vi "sequential on_off.vi"() -> ()   [LabVIEW 2018]
doc: "Manually blink and LED attached to a digital output channel of a LINX device by clicking and LED control in LabVIEW."
uses:
  <vilib>/MakerHub/LINX/Public/Peripherals/Digital/Digital Write 1 Chan.vi
  <vilib>/MakerHub/LINX/Public/Peripherals/Digital/Digital Write N Chans.vi
  <vilib>/MakerHub/LINX/Private/Local IO/LinxDigitalWrite.vi
  <vilib>/MakerHub/LINX/Public/Utilities/Check Channel.vi
  <vilib>/MakerHub/LINX/Public/Utilities/Open Serial.vi
  <vilib>/MakerHub/LINX/Private/Utilties/Generate Error.vi
  <vilib>/MakerHub/LINX/LMH-LINX.lvlib
panel:
  out "ch_4":bool
  out "ch_3":bool
  out "ch_2":bool
  out "ch_1":bool
  in  "Delay (ms)":dbl
  in  "Chnl_4":bool
  in  "Chnl_3":bool
  in  "Chnl_2":bool
  in  "Chnl_1":bool
  in  "Reset valves":bool
  out "id_8":bool
  out "id_7":bool
  out "id_6":bool
  out "id_5":bool
  out "id_4":bool
  out "id_3":bool
  out "id_2":bool
  out "id_1":bool
  in  "stop":bool
  in  "Valve 8":bool
  in  "Valve 7":bool
  in  "Valve 6":bool
  in  "Valve 5":bool
  in  "Valve 4":bool
  in  "Valve 3":bool
  in  "Valve 2":bool
  in  "Valve_1":bool
  in  "Serial Port":refnum<visa-resource-name>
  # "Manual Control:"
  # "LINX Device Settings"
  # "Sequential Control:"
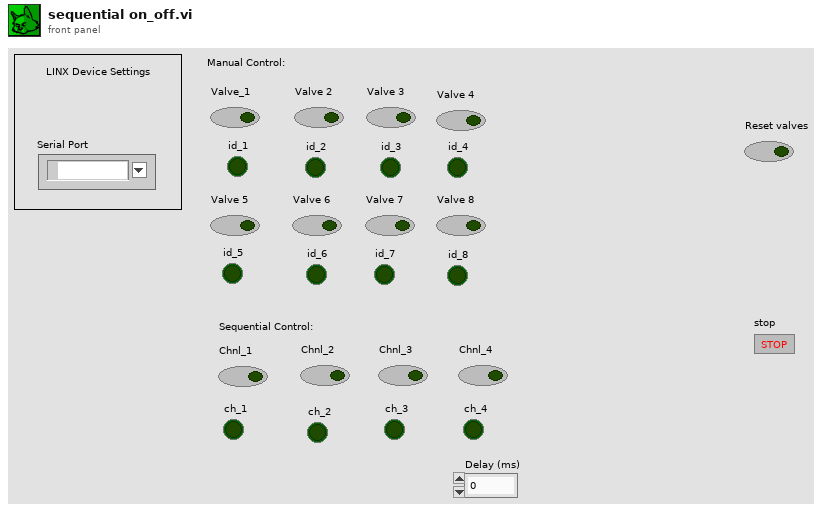
[diagram p1: front panel]
types:
  T1 = typedef "LMH-LINX.lvlib/LINX Ref.ctl" = cluster{"IO":T2, "Interface":T3, "LINX Device Config":T4}
  T2 = typedef "LMH-LINX.lvlib/Platform.ctl" = enum16{"Remote", "Local"}
  T3 = typedef "LMH-LINX.lvlib/Interface.ctl" = enum16{"Serial", "TCP"}
  T4 = typedef "LMH-LINX.lvlib/Device.lvlib/LINX Device Config.ctl" = cluster{"Interface":T3, "COM Port":refnum<visa-resource-name>, "TCP Configuration":T5, "Device Family":u8, "Device ID":u8, "Device Name":string, "TCP Ref":refnum<k5>, "Channels":T6}
  T5 = typedef "LMH-LINX.lvlib/Device.lvlib/TCP Config.ctl" = cluster{"IP Address":string, "Port":u16}
  T6 = typedef "LMH-LINX.lvlib/Channels.ctl" = cluster{"DI":u8[], "DO":u8[], "AI":u8[], "AO":u8[], "PWM":u8[], "QE":u8[], "UART":u8[], "I2C 2":u8[], "SPI":u8[], "CAN":u8[], "Servo":u8[], "AI Ref (V)":dbl, "AI Resolution (Bits)":u8, "AO Ref (V)":dbl, "AO Resolution (Bits)":u8}
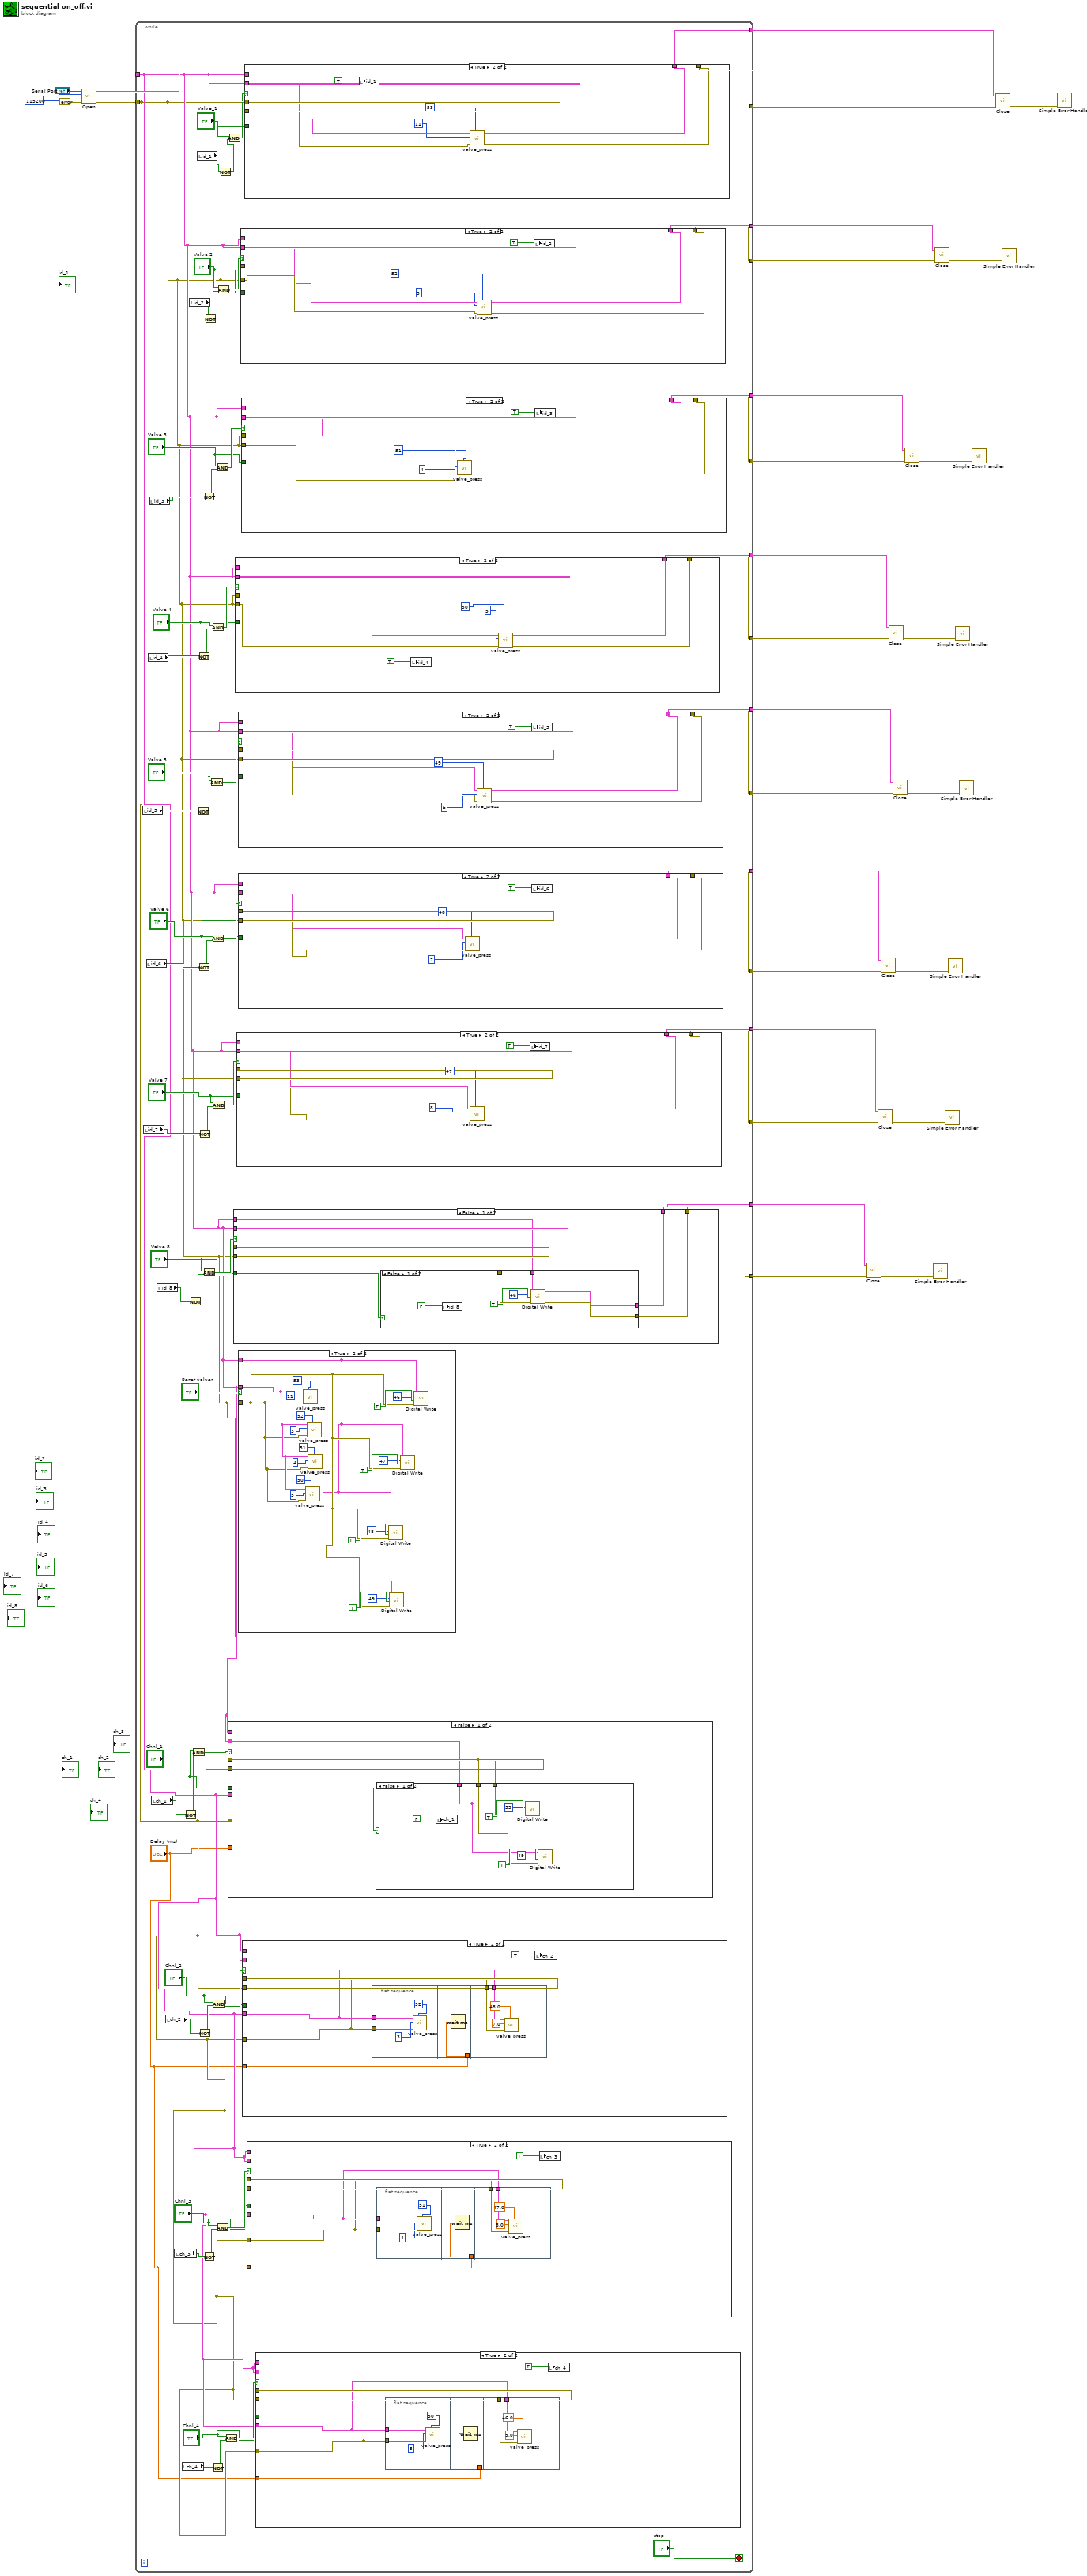
[diagram p0: block diagram]
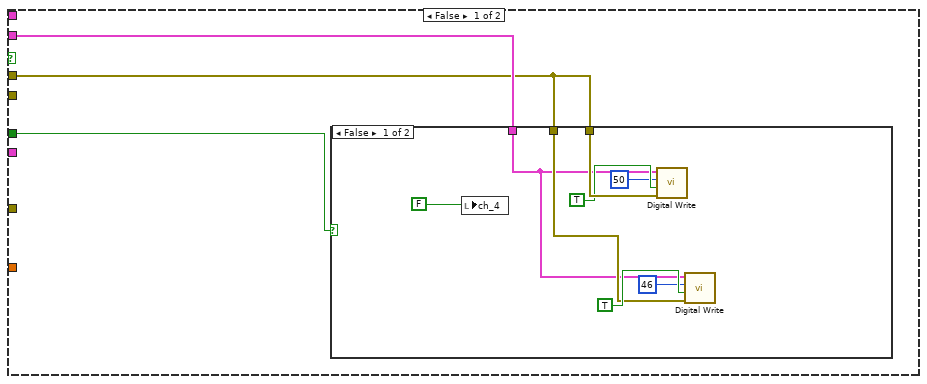
[diagram p2: hidden frame]
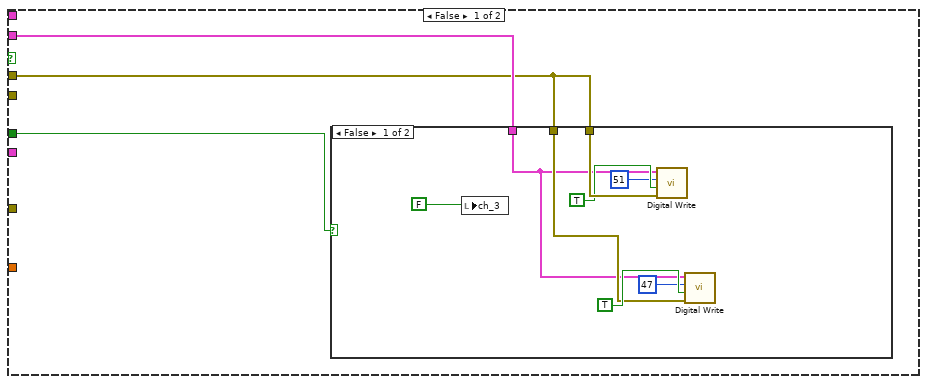
[diagram p4: hidden frame]
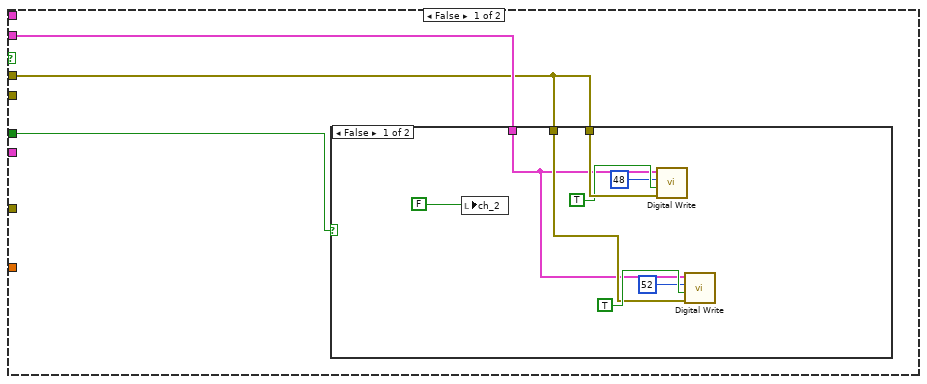
[diagram p6: hidden frame]
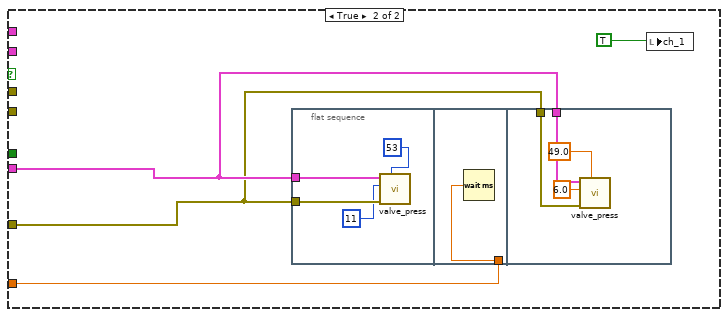
[diagram p9: hidden frame]
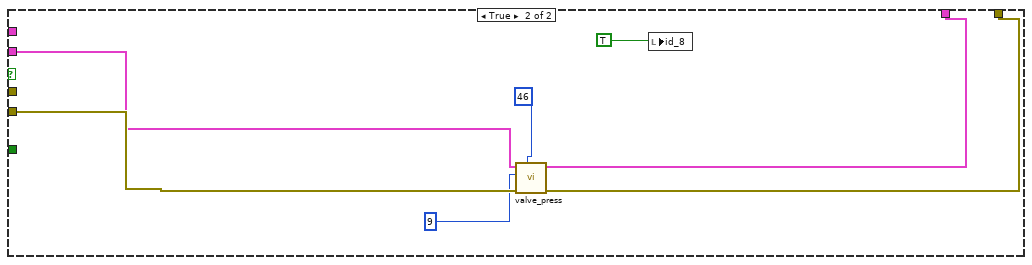
[diagram p12: hidden frame]
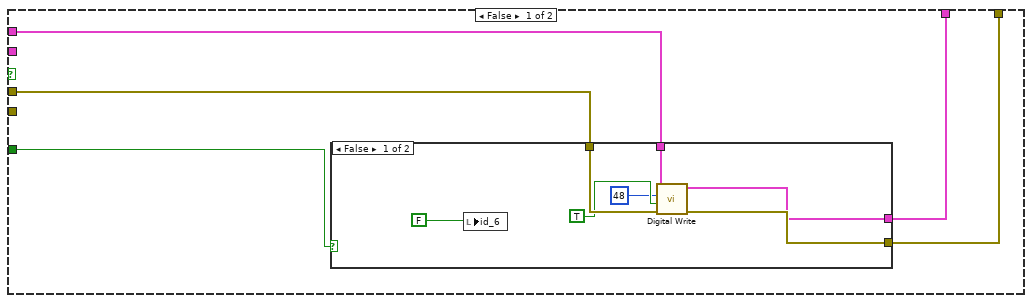
[diagram p13: hidden frame]
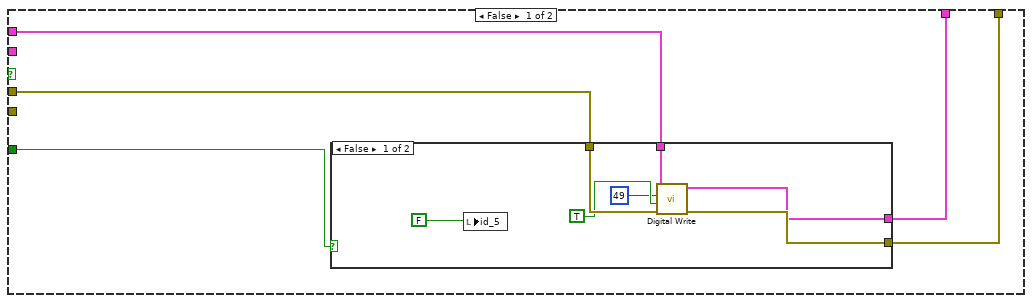
[diagram p15: hidden frame]
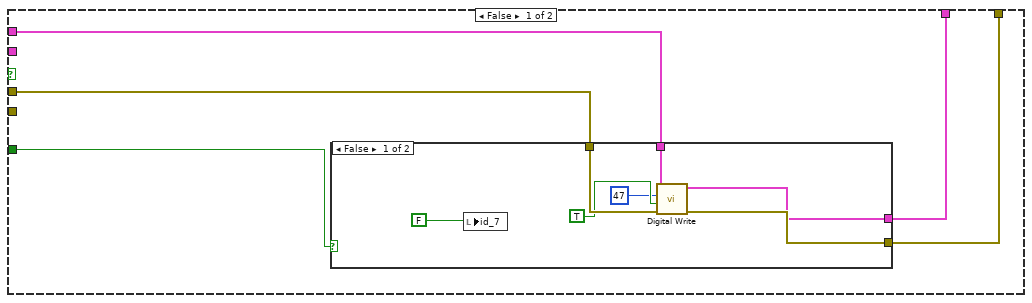
[diagram p17: hidden frame]
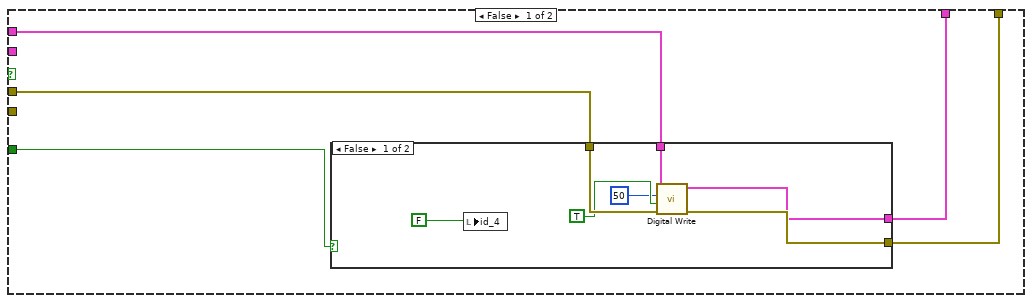
[diagram p19: hidden frame]
diagram:
  n1 = call-poly <vilib>:"Open.vi"("Error In"=errorcluster {"status"=FALSE, "code"=0, "source"=""}, "Baud Rate Override"=u32 115200, "Serial Port"="Serial Port") -> ("Error Out"=w25:errorcluster, "LINX Resource"=w26:T1)  [unwired: 6 in, 1 out]
  n2 = while {
    tunnel: w26 -> [w35]
    tunnel: w25 -> [w34]
    tunnel: [w97] -> w24
    tunnel: [w96] -> w23
    tunnel: [w92] -> w21
    tunnel: [w91] -> w14
    tunnel: [w90] -> w13
    tunnel: [w89] -> w12
    tunnel: [w88] -> w11
    tunnel: [w87] -> w10
    tunnel: [w86] -> w9
    tunnel: [w85] -> w8
    tunnel: [w84] -> w7
    tunnel: [w83] -> w6
    tunnel: [w82] -> w5
    tunnel: [w81] -> w4
    tunnel: [w50] -> w3
    tunnel: [w73] -> w2
    stop <- "stop" stop-if-true
    n3 = local read "id_5"() -> (w68:bool)
    n4 = local read "id_7"() -> (w66:bool)
    n5 = local read "id_6"() -> (w67:bool)
    n6 = local read "id_4"() -> (w69:bool)
    n7 = local read "id_3"() -> (w70:bool)
    n8 = local read "ch_1"() -> (w49:bool)
    n9 = local read "id_8"() -> (w65:bool)
    n10 = local read "ch_2"() -> (w45:bool)
    n11 = local read "ch_3"() -> (w38:bool)
    n12 = local read "ch_4"() -> (w32:bool)
    n13 = Not(x=w49) -> (.not. x?=w48:bool)
    n14 = Not(x=w65) -> (.not. x?=w64:bool)
    n15 = local read "id_2"() -> (w78:bool)
    n16 = And(x="Chnl_1", y=w48) -> (x .and. y?=w47:bool)
    n17 = Not(x=w68) -> (.not. x?=w58:bool)
    n18 = local read "id_1"() -> (w94:bool)
    n19 = Not(x=w69) -> (.not. x?=w72:bool)
    n20 = Not(x=w67) -> (.not. x?=w60:bool)
    n21 = Not(x=w66) -> (.not. x?=w62:bool)
    n22 = Not(x=w45) -> (.not. x?=w44:bool)
    n23 = Not(x=w70) -> (.not. x?=w76:bool)
    n24 = And(x="Valve 8", y=w64) -> (x .and. y?=w63:bool)
    n25 = Not(x=w38) -> (.not. x?=w41:bool)
    n26 = Not(x=w78) -> (.not. x?=w79:bool)
    n27 = And(x="Valve 5", y=w58) -> (x .and. y?=w57:bool)
    n28 = And(x="Valve 4", y=w72) -> (x .and. y?=w71:bool)
    n29 = And(x="Valve 6", y=w60) -> (x .and. y?=w59:bool)
    n30 = Not(x=w32) -> (.not. x?=w37:bool)
    n31 = And(x="Valve 7", y=w62) -> (x .and. y?=w61:bool)
    n32 = And(x="Chnl_2", y=w44) -> (x .and. y?=w43:bool)
    n33 = And(x="Valve 3", y=w76) -> (x .and. y?=w75:bool)
    n34 = And(x="Chnl_3", y=w41) -> (x .and. y?=w40:bool)
    n35 = And(x="Valve 2", y=w79) -> (x .and. y?=w80:bool)
    n36 = Not(x=w94) -> (.not. x?=w93:bool)
    n37 = And(x="Chnl_4", y=w37) -> (x .and. y?=w36:bool)
    n38 = And(x="Valve_1", y=w93) -> (x .and. y?=w95:bool)
    n39 = case shown="False" w47 {
      tunnel: w35 -> [w172 _]
      tunnel: w34 -> [_ _]
      tunnel: "Chnl_1" -> [w173 _]
      tunnel: w34 -> [w171 _]
      tunnel: w35 -> [_ _]
      tunnel: w34 -> [_ w183]
      tunnel: w35 -> [_ w184]
      tunnel: "Delay (ms)" -> [_ w185]
      frame False {
        n40 = case shown="False" w173 {
          tunnel: w171 -> [w181 _]
          tunnel: w172 -> [w174 _]
          tunnel: w171 -> [w175 _]
          frame False {
            n41 = local write "ch_1"(FALSE) -> ()
            n42 = call-poly <vilib>:"Digital Write.vi"("Error In"=w181, "Output Value"=TRUE, "DO Channel"=u8 53, "LINX Resource"=w174) -> ()  [unwired: 6 in, 2 out]
            n43 = call-poly <vilib>:"Digital Write.vi"("Error In"=w175, "Output Value"=TRUE, "DO Channel"=u8 49, "LINX Resource"=w174) -> ()  [unwired: 6 in, 2 out]
          }
          frame True {
          }
        }
      }
      frame True {
        n44 = flat-sequence {
          tunnel: w183 -> [w188]
          tunnel: w184 -> [w186]
          tunnel: w185 -> [w190]
          tunnel: w184 -> [w194]
          tunnel: w183 -> [w193]
          frame #0 {
            n45 = call "valve_press.vi"("power"=53, "error in (no error)"=w188, "trigger"=11, "LINX Resource in"=w186) -> ()  [unwired: 6 in, 2 out]
          }
          frame #1 {
            n46 = Wait (ms)(milliseconds to wait=w190) -> ()  [unwired: 1 out]
          }
          frame #2 {
            n47 = call "valve_press.vi"("power"=49.0, "error in (no error)"=w193, "trigger"=6.0, "LINX Resource in"=w194) -> ()  [unwired: 6 in, 2 out]
          }
        }
        n48 = local write "ch_1"(TRUE) -> ()
      }
    }
    n49 = case shown="False" w63 {
      tunnel: w35 -> [_ w232]
      tunnel: w34 -> [_ w233]
      tunnel: [w214 w231] -> w50
      tunnel: [w215 w230] -> w73
      tunnel: "Valve 8" -> [w218 _]
      tunnel: w34 -> [w217 _]
      tunnel: w35 -> [w216 _]
      frame False {
        n50 = case shown="False" w218 {
          tunnel: w217 -> [w224 w226]
          tunnel: w216 -> [w221 w227]
          tunnel: [w220 w226] -> w215
          tunnel: [w219 w227] -> w214
          frame False {
            n51 = local write "id_8"(FALSE) -> ()
            n52 = call-poly <vilib>:"Digital Write.vi"("Error In"=w224, "Output Value"=TRUE, "DO Channel"=u8 46, "LINX Resource"=w221) -> ("Error Out"=w220:errorcluster, "LINX Resource"=w219:T1)  [unwired: 6 in]
          }
          frame True {
          }
        }
      }
      frame True {
        n53 = call "valve_press.vi"("power"=46, "error in (no error)"=w233, "trigger"=9, "LINX Resource in"=w232) -> ("error out"=w230:errorcluster, "LINX Resource out"=w231:T1)  [unwired: 6 in]
        n54 = local write "id_8"(TRUE) -> ()
      }
    }
    n55 = case shown="True" w71 {
      tunnel: w35 -> [_ w318]
      tunnel: w34 -> [_ w317]
      tunnel: [w298 w316] -> w88
      tunnel: [w299 w315] -> w84
      tunnel: "Valve 4" -> [w302 _]
      tunnel: w34 -> [w301 _]
      tunnel: w35 -> [w300 _]
      frame False {
        n56 = case shown="False" w302 {
          tunnel: w301 -> [w308 w310]
          tunnel: w300 -> [w305 w311]
          tunnel: [w304 w310] -> w299
          tunnel: [w303 w311] -> w298
          frame False {
            n57 = local write "id_4"(FALSE) -> ()
            n58 = call-poly <vilib>:"Digital Write.vi"("Error In"=w308, "Output Value"=TRUE, "DO Channel"=u8 50, "LINX Resource"=w305) -> ("Error Out"=w304:errorcluster, "LINX Resource"=w303:T1)  [unwired: 6 in]
          }
          frame True {
          }
        }
      }
      frame True {
        n59 = local write "id_4"(TRUE) -> ()
        n60 = call "valve_press.vi"("power"=50, "error in (no error)"=w317, "trigger"=5, "LINX Resource in"=w318) -> ("error out"=w315:errorcluster, "LINX Resource out"=w316:T1)  [unwired: 6 in]
      }
    }
    n61 = case shown="True" w61 {
      tunnel: w35 -> [_ w296]
      tunnel: w34 -> [_ w295]
      tunnel: [w277 w293] -> w91
      tunnel: [w278 w294] -> w81
      tunnel: "Valve 7" -> [w281 _]
      tunnel: w34 -> [w280 _]
      tunnel: w35 -> [w279 _]
      frame False {
        n62 = case shown="False" w281 {
          tunnel: w280 -> [w287 w289]
          tunnel: w279 -> [w284 w290]
          tunnel: [w283 w289] -> w278
          tunnel: [w282 w290] -> w277
          frame False {
            n63 = local write "id_7"(FALSE) -> ()
            n64 = call-poly <vilib>:"Digital Write.vi"("Error In"=w287, "Output Value"=TRUE, "DO Channel"=u8 47, "LINX Resource"=w284) -> ("Error Out"=w283:errorcluster, "LINX Resource"=w282:T1)  [unwired: 6 in]
          }
          frame True {
          }
        }
      }
      frame True {
        n65 = call "valve_press.vi"("power"=47, "error in (no error)"=w295, "trigger"=8, "LINX Resource in"=w296) -> ("error out"=w294:errorcluster, "LINX Resource out"=w293:T1)  [unwired: 6 in]
        n66 = local write "id_7"(TRUE) -> ()
      }
    }
    n67 = case shown="True" w57 {
      tunnel: w35 -> [_ w272]
      tunnel: w34 -> [_ w273]
      tunnel: [w256 w275] -> w89
      tunnel: [w257 w274] -> w83
      tunnel: "Valve 5" -> [w260 _]
      tunnel: w34 -> [w259 _]
      tunnel: w35 -> [w258 _]
      frame False {
        n68 = case shown="False" w260 {
          tunnel: w259 -> [w266 w268]
          tunnel: w258 -> [w263 w269]
          tunnel: [w262 w268] -> w257
          tunnel: [w261 w269] -> w256
          frame False {
            n69 = local write "id_5"(FALSE) -> ()
            n70 = call-poly <vilib>:"Digital Write.vi"("Error In"=w266, "Output Value"=TRUE, "DO Channel"=u8 49, "LINX Resource"=w263) -> ("Error Out"=w262:errorcluster, "LINX Resource"=w261:T1)  [unwired: 6 in]
          }
          frame True {
          }
        }
      }
      frame True {
        n71 = call "valve_press.vi"("power"=49, "error in (no error)"=w273, "trigger"=6, "LINX Resource in"=w272) -> ("error out"=w274:errorcluster, "LINX Resource out"=w275:T1)  [unwired: 6 in]
        n72 = local write "id_5"(TRUE) -> ()
      }
    }
    n73 = case shown="True" w59 {
      tunnel: w35 -> [_ w253]
      tunnel: w34 -> [_ w254]
      tunnel: [w235 w252] -> w90
      tunnel: [w236 w251] -> w82
      tunnel: "Valve 6" -> [w239 _]
      tunnel: w34 -> [w238 _]
      tunnel: w35 -> [w237 _]
      frame False {
        n74 = case shown="False" w239 {
          tunnel: w238 -> [w245 w247]
          tunnel: w237 -> [w242 w248]
          tunnel: [w241 w247] -> w236
          tunnel: [w240 w248] -> w235
          frame False {
            n75 = local write "id_6"(FALSE) -> ()
            n76 = call-poly <vilib>:"Digital Write.vi"("Error In"=w245, "Output Value"=TRUE, "DO Channel"=u8 48, "LINX Resource"=w242) -> ("Error Out"=w241:errorcluster, "LINX Resource"=w240:T1)  [unwired: 6 in]
          }
          frame True {
          }
        }
      }
      frame True {
        n77 = call "valve_press.vi"("power"=48, "error in (no error)"=w254, "trigger"=7, "LINX Resource in"=w253) -> ("error out"=w251:errorcluster, "LINX Resource out"=w252:T1)  [unwired: 6 in]
        n78 = local write "id_6"(TRUE) -> ()
      }
    }
    n79 = case shown="True" "Reset valves" {
      tunnel: w35 -> [_ w213]
      tunnel: w34 -> [_ w196]
      tunnel: w35 -> [_ w195]
      frame False {
      }
      frame True {
        n80 = call "valve_press.vi"("power"=53, "error in (no error)"=w196, "trigger"=11, "LINX Resource in"=w213) -> ()  [unwired: 6 in, 2 out]
        n81 = call "valve_press.vi"("power"=50, "error in (no error)"=w196, "trigger"=5, "LINX Resource in"=w213) -> ()  [unwired: 6 in, 2 out]
        n82 = call "valve_press.vi"("power"=52, "error in (no error)"=w196, "trigger"=3, "LINX Resource in"=w213) -> ()  [unwired: 6 in, 2 out]
        n83 = call "valve_press.vi"("power"=51, "error in (no error)"=w196, "trigger"=4, "LINX Resource in"=w213) -> ()  [unwired: 6 in, 2 out]
        n84 = call-poly <vilib>:"Digital Write.vi"("Error In"=w196, "Output Value"=TRUE, "DO Channel"=u8 48, "LINX Resource"=w195) -> ()  [unwired: 6 in, 2 out]
        n85 = call-poly <vilib>:"Digital Write.vi"("Error In"=w196, "Output Value"=TRUE, "DO Channel"=u8 49, "LINX Resource"=w195) -> ()  [unwired: 6 in, 2 out]
        n86 = call-poly <vilib>:"Digital Write.vi"("Error In"=w196, "Output Value"=TRUE, "DO Channel"=u8 47, "LINX Resource"=w195) -> ()  [unwired: 6 in, 2 out]
        n87 = call-poly <vilib>:"Digital Write.vi"("Error In"=w196, "Output Value"=TRUE, "DO Channel"=u8 46, "LINX Resource"=w195) -> ()  [unwired: 6 in, 2 out]
      }
    }
    n88 = case shown="True" w80 {
      tunnel: w35 -> [_ w358]
      tunnel: [w340 w357] -> w92
      tunnel: [w341 w356] -> w86
      tunnel: "Valve 2" -> [w344 _]
      tunnel: w34 -> [w343 _]
      tunnel: w35 -> [w342 _]
      tunnel: w34 -> [_ w359]
      frame False {
        n89 = case shown="False" w344 {
          tunnel: w343 -> [w350 w352]
          tunnel: w342 -> [w347 w353]
          tunnel: [w346 w352] -> w341
          tunnel: [w345 w353] -> w340
          frame False {
            n90 = local write "id_2"(FALSE) -> ()
            n91 = call-poly <vilib>:"Digital Write.vi"("Error In"=w350, "Output Value"=TRUE, "DO Channel"=u8 52, "LINX Resource"=w347) -> ("Error Out"=w346:errorcluster, "LINX Resource"=w345:T1)  [unwired: 6 in]
          }
          frame True {
          }
        }
      }
      frame True {
        n92 = call "valve_press.vi"("power"=52, "error in (no error)"=w359, "trigger"=3, "LINX Resource in"=w358) -> ("error out"=w356:errorcluster, "LINX Resource out"=w357:T1)  [unwired: 6 in]
        n93 = local write "id_2"(TRUE) -> ()
      }
    }
    n94 = case shown="True" w75 {
      tunnel: w35 -> [_ w337]
      tunnel: w34 -> [_ w338]
      tunnel: [w319 w336] -> w87
      tunnel: [w320 w335] -> w85
      tunnel: "Valve 3" -> [w323 _]
      tunnel: w34 -> [w322 _]
      tunnel: w35 -> [w321 _]
      frame False {
        n95 = case shown="False" w323 {
          tunnel: w322 -> [w329 w331]
          tunnel: w321 -> [w326 w332]
          tunnel: [w325 w331] -> w320
          tunnel: [w324 w332] -> w319
          frame False {
            n96 = local write "id_3"(FALSE) -> ()
            n97 = call-poly <vilib>:"Digital Write.vi"("Error In"=w329, "Output Value"=TRUE, "DO Channel"=u8 51, "LINX Resource"=w326) -> ("Error Out"=w325:errorcluster, "LINX Resource"=w324:T1)  [unwired: 6 in]
          }
          frame True {
          }
        }
      }
      frame True {
        n98 = call "valve_press.vi"("power"=51, "error in (no error)"=w338, "trigger"=4, "LINX Resource in"=w337) -> ("error out"=w335:errorcluster, "LINX Resource out"=w336:T1)  [unwired: 6 in]
        n99 = local write "id_3"(TRUE) -> ()
      }
    }
    n100 = case shown="True" w43 {
      tunnel: w35 -> [w148 _]
      tunnel: w34 -> [_ _]
      tunnel: "Chnl_2" -> [w149 _]
      tunnel: w34 -> [w147 _]
      tunnel: w35 -> [_ _]
      tunnel: w34 -> [_ w159]
      tunnel: w35 -> [_ w160]
      tunnel: "Delay (ms)" -> [_ w161]
      frame False {
        n101 = case shown="False" w149 {
          tunnel: w147 -> [w157 _]
          tunnel: w148 -> [w150 _]
          tunnel: w147 -> [w151 _]
          frame False {
            n102 = local write "ch_2"(FALSE) -> ()
            n103 = call-poly <vilib>:"Digital Write.vi"("Error In"=w157, "Output Value"=TRUE, "DO Channel"=u8 48, "LINX Resource"=w150) -> ()  [unwired: 6 in, 2 out]
            n104 = call-poly <vilib>:"Digital Write.vi"("Error In"=w151, "Output Value"=TRUE, "DO Channel"=u8 52, "LINX Resource"=w150) -> ()  [unwired: 6 in, 2 out]
          }
          frame True {
          }
        }
      }
      frame True {
        n105 = flat-sequence {
          tunnel: w159 -> [w164]
          tunnel: w160 -> [w162]
          tunnel: w161 -> [w166]
          tunnel: w160 -> [w170]
          tunnel: w159 -> [w169]
          frame #0 {
            n106 = call "valve_press.vi"("power"=52, "error in (no error)"=w164, "trigger"=3, "LINX Resource in"=w162) -> ()  [unwired: 6 in, 2 out]
          }
          frame #1 {
            n107 = Wait (ms)(milliseconds to wait=w166) -> ()  [unwired: 1 out]
          }
          frame #2 {
            n108 = call "valve_press.vi"("power"=48.0, "error in (no error)"=w169, "trigger"=7.0, "LINX Resource in"=w170) -> ()  [unwired: 6 in, 2 out]
          }
        }
        n109 = local write "ch_2"(TRUE) -> ()
      }
    }
    n110 = case shown="True" w95 {
      tunnel: w35 -> [_ w380]
      tunnel: w34 -> [_ w381]
      tunnel: [w362 w379] -> w97
      tunnel: [w363 w378] -> w96
      tunnel: w34 -> [w365 _]
      tunnel: w35 -> [w364 _]
      tunnel: "Valve_1" -> [w361 _]
      frame False {
        n111 = case shown="False" w361 {
          tunnel: w365 -> [w371 w373]
          tunnel: w364 -> [w368 w374]
          tunnel: [w367 w373] -> w363
          tunnel: [w366 w374] -> w362
          frame False {
            n112 = local write "id_1"(FALSE) -> ()
            n113 = call-poly <vilib>:"Digital Write.vi"("Error In"=w371, "Output Value"=TRUE, "DO Channel"=u8 53, "LINX Resource"=w368) -> ("Error Out"=w367:errorcluster, "LINX Resource"=w366:T1)  [unwired: 6 in]
          }
          frame True {
          }
        }
      }
      frame True {
        n114 = local write "id_1"(TRUE) -> ()
        n115 = call "valve_press.vi"("power"=53, "error in (no error)"=w381, "trigger"=11, "LINX Resource in"=w380) -> ("error out"=w378:errorcluster, "LINX Resource out"=w379:T1)  [unwired: 6 in]
      }
    }
    n116 = case shown="True" w40 {
      tunnel: w35 -> [w124 _]
      tunnel: w34 -> [_ _]
      tunnel: "Chnl_3" -> [w125 _]
      tunnel: w34 -> [w123 _]
      tunnel: w35 -> [_ _]
      tunnel: w34 -> [_ w135]
      tunnel: w35 -> [_ w136]
      tunnel: "Delay (ms)" -> [_ w137]
      frame False {
        n117 = case shown="False" w125 {
          tunnel: w123 -> [w133 _]
          tunnel: w124 -> [w126 _]
          tunnel: w123 -> [w127 _]
          frame False {
            n118 = local write "ch_3"(FALSE) -> ()
            n119 = call-poly <vilib>:"Digital Write.vi"("Error In"=w133, "Output Value"=TRUE, "DO Channel"=u8 51, "LINX Resource"=w126) -> ()  [unwired: 6 in, 2 out]
            n120 = call-poly <vilib>:"Digital Write.vi"("Error In"=w127, "Output Value"=TRUE, "DO Channel"=u8 47, "LINX Resource"=w126) -> ()  [unwired: 6 in, 2 out]
          }
          frame True {
          }
        }
      }
      frame True {
        n121 = flat-sequence {
          tunnel: w135 -> [w140]
          tunnel: w136 -> [w138]
          tunnel: w137 -> [w142]
          tunnel: w136 -> [w146]
          tunnel: w135 -> [w145]
          frame #0 {
            n122 = call "valve_press.vi"("power"=51, "error in (no error)"=w140, "trigger"=4, "LINX Resource in"=w138) -> ()  [unwired: 6 in, 2 out]
          }
          frame #1 {
            n123 = Wait (ms)(milliseconds to wait=w142) -> ()  [unwired: 1 out]
          }
          frame #2 {
            n124 = call "valve_press.vi"("power"=47.0, "error in (no error)"=w145, "trigger"=8.0, "LINX Resource in"=w146) -> ()  [unwired: 6 in, 2 out]
          }
        }
        n125 = local write "ch_3"(TRUE) -> ()
      }
    }
    n126 = case shown="True" w36 {
      tunnel: w35 -> [w100 _]
      tunnel: w34 -> [_ _]
      tunnel: "Chnl_4" -> [w101 _]
      tunnel: w34 -> [w99 _]
      tunnel: w35 -> [_ _]
      tunnel: w34 -> [_ w111]
      tunnel: w35 -> [_ w112]
      tunnel: "Delay (ms)" -> [_ w113]
      frame False {
        n127 = case shown="False" w101 {
          tunnel: w99 -> [w109 _]
          tunnel: w100 -> [w102 _]
          tunnel: w99 -> [w103 _]
          frame False {
            n128 = local write "ch_4"(FALSE) -> ()
            n129 = call-poly <vilib>:"Digital Write.vi"("Error In"=w109, "Output Value"=TRUE, "DO Channel"=u8 50, "LINX Resource"=w102) -> ()  [unwired: 6 in, 2 out]
            n130 = call-poly <vilib>:"Digital Write.vi"("Error In"=w103, "Output Value"=TRUE, "DO Channel"=u8 46, "LINX Resource"=w102) -> ()  [unwired: 6 in, 2 out]
          }
          frame True {
          }
        }
      }
      frame True {
        n131 = flat-sequence {
          tunnel: w111 -> [w116]
          tunnel: w112 -> [w114]
          tunnel: w113 -> [w118]
          tunnel: w112 -> [w122]
          tunnel: w111 -> [w121]
          frame #0 {
            n132 = call "valve_press.vi"("power"=50, "error in (no error)"=w116, "trigger"=5, "LINX Resource in"=w114) -> ()  [unwired: 6 in, 2 out]
          }
          frame #1 {
            n133 = Wait (ms)(milliseconds to wait=w118) -> ()  [unwired: 1 out]
          }
          frame #2 {
            n134 = call "valve_press.vi"("power"=46.0, "error in (no error)"=w121, "trigger"=9.0, "LINX Resource in"=w122) -> ()  [unwired: 6 in, 2 out]
          }
        }
        n135 = local write "ch_4"(TRUE) -> ()
      }
    }
  }
  n136 = call <vilib>:"Close.vi"("Error In"=w2, "LINX Resource"=w3) -> ("Error Out"=w1:errorcluster)  [unwired: 9 in]
  n137 = call <vilib>:"Close.vi"("Error In"=w4, "LINX Resource"=w14) -> ("Error Out"=w15:errorcluster)  [unwired: 9 in]
  n138 = call <vilib>:"Close.vi"("Error In"=w5, "LINX Resource"=w13) -> ("Error Out"=w16:errorcluster)  [unwired: 9 in]
  n139 = call <vilib>:"Close.vi"("Error In"=w7, "LINX Resource"=w11) -> ("Error Out"=w18:errorcluster)  [unwired: 9 in]
  n140 = call <vilib>:"Close.vi"("Error In"=w6, "LINX Resource"=w12) -> ("Error Out"=w17:errorcluster)  [unwired: 9 in]
  n141 = call <vilib>:"Close.vi"("Error In"=w8, "LINX Resource"=w10) -> ("Error Out"=w19:errorcluster)  [unwired: 9 in]
  n142 = call <vilib>:"Simple Error Handler.vi"("error in (no error)"=w1) -> ()  [unwired: 4 in, 5 out]
  n143 = call <vilib>:"Close.vi"("Error In"=w9, "LINX Resource"=w21) -> ("Error Out"=w20:errorcluster)  [unwired: 9 in]
  n144 = call <vilib>:"Simple Error Handler.vi"("error in (no error)"=w15) -> ()  [unwired: 4 in, 5 out]
  n145 = call <vilib>:"Simple Error Handler.vi"("error in (no error)"=w16) -> ()  [unwired: 4 in, 5 out]
  n146 = call <vilib>:"Simple Error Handler.vi"("error in (no error)"=w18) -> ()  [unwired: 4 in, 5 out]
  n147 = call <vilib>:"Simple Error Handler.vi"("error in (no error)"=w17) -> ()  [unwired: 4 in, 5 out]
  n148 = call <vilib>:"Simple Error Handler.vi"("error in (no error)"=w19) -> ()  [unwired: 4 in, 5 out]
  n149 = call <vilib>:"Close.vi"("Error In"=w23, "LINX Resource"=w24) -> ("Error Out"=w28:errorcluster)  [unwired: 9 in]
  n150 = call <vilib>:"Simple Error Handler.vi"("error in (no error)"=w20) -> ()  [unwired: 4 in, 5 out]
  n151 = call <vilib>:"Simple Error Handler.vi"("error in (no error)"=w28) -> ()  [unwired: 4 in, 5 out]
